vi "Simple Reader.vi"(8 "error in (no error)":errorcluster, 11 "Keithley 622x2182 Driver in":refnum<class "Keithley 622x2182 Driver.lvclass">) -> (0 "error out":errorcluster, 2 "Signals":dbl[](array[numeric]), 3 "Keithley 622x2182 Driver out":refnum<class "Keithley 622x2182 Driver.lvclass">)   [LabVIEW 2021, in "Keithley 622x2182 Driver.lvclass"]
uses:
  Keithley 622x2182 Driver.lvclass
  C:/Git/NHMFL_Core/Libraries/Instruments/VISA Instrument/VISA Instrument.lvclass
  VISA Instrument/VISA Instrument.lvclass/VISA Instrument.ctl
  VISA Instrument/Read VISA resource.vi
  VISA Instrument/Write VISA resource.vi
panel:
  out "array":dbl[][](array[numeric])
  out "read buffer":string
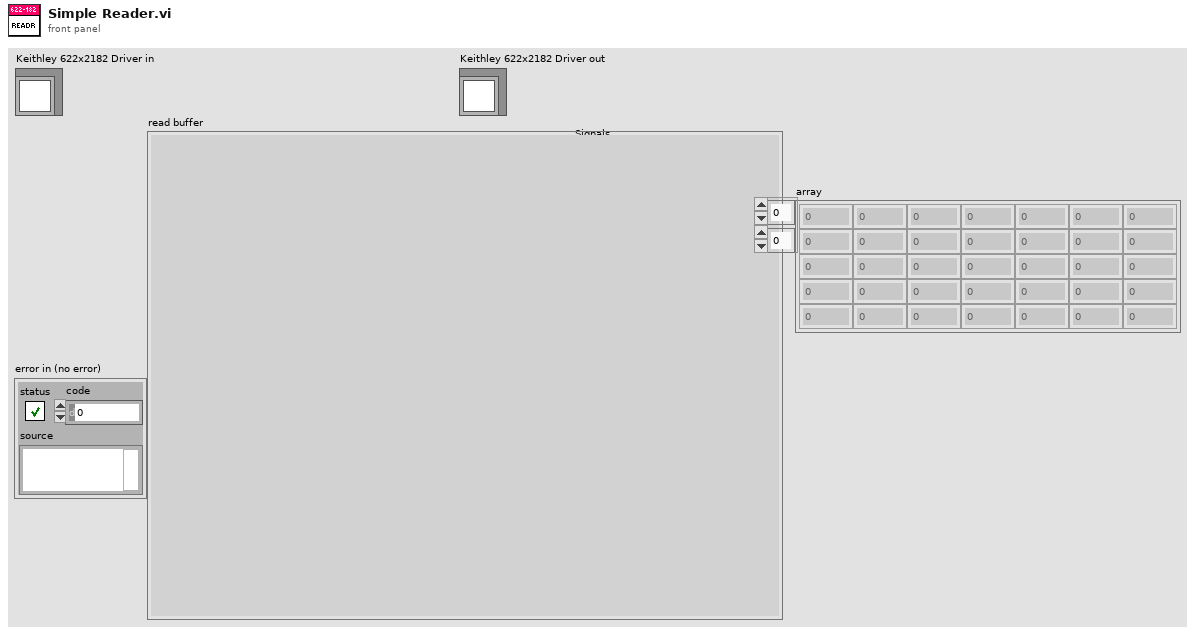
[diagram p1: front panel]
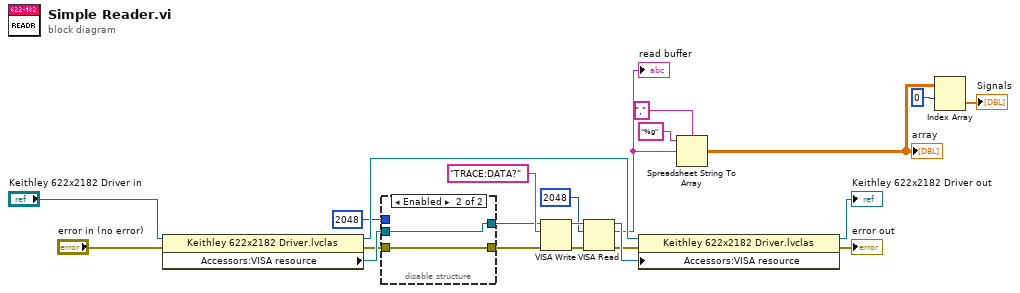
[diagram p0: block diagram]
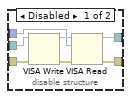
[diagram p2: hidden frame]
diagram:
  n1 = property class="Keithley 622x2182 Driver.lvclas"(reference="Keithley 622x2182 Driver in", error in="error in (no error)") -> (reference out=w13:refnum<class "Keithley 622x2182 Driver.lvclass">, error out=w2:errorcluster, "Accessors:VISA resource"=w3:refnum<visa-resource-name>)
  n2 = disable-structure shown="Enabled" {
    disable-tunnel: u32 2048 ("byte count") -> [w29 _]
    disable-tunnel: [w26 w31] -> w4
    disable-tunnel: w3 -> [w25 w30]
    disable-tunnel: w2 -> [w24 w31]
    disable-tunnel: [w23 w30] -> w1
    frame Disabled {
      n3 = VISA Write(VISA resource name=w25, error in (no error)=w24) -> (VISA resource name out=w28:refnum<visa-resource-name>, error out=w27:errorcluster)  [unwired: 1 in, 1 out]
      n4 = VISA Read(VISA resource name=w28, byte count=w29, error in (no error)=w27) -> (VISA resource name out=w23:refnum<visa-resource-name>, error out=w26:errorcluster)  [unwired: 2 out]
    }
    frame Enabled {
    }
  }
  n5 = VISA Write(VISA resource name=w1, write buffer="TRACE:DATA?", error in (no error)=w4) -> (VISA resource name out=w16:refnum<visa-resource-name>, error out=w17:errorcluster)  [unwired: 1 out]
  n6 = VISA Read(VISA resource name=w16, byte count=u32 2048, error in (no error)=w17) -> (VISA resource name out=w14:refnum<visa-resource-name>, read buffer=w11:string, error out=w12:errorcluster)  [unwired: 1 out]
  "read buffer" <- w11
  n7 = property class="Keithley 622x2182 Driver.lvclas"(reference=w13, error in=w12, "Accessors:VISA resource"=w14) -> (reference out=→"Keithley 622x2182 Driver out":refnum<class "Keithley 622x2182 Driver.lvclass">, error out=→"error out":errorcluster)
  n8 = Spreadsheet String To Array(delimiter (Tab)=",", format string="%g", spreadsheet string=w11) -> (array=w8:dbl[][])  [unwired: 1 in]
  "array" <- w8
  n9 = Index Array(array=w8, index (row)=0) -> (element=→"Signals":dbl[])  [unwired: 1 in]
